vi "UI_update_Zone_indicator_params.vi"(8 "error in (no error)":errorcluster, 10 "Geometry params in":T1 {"Cage diameter, mm" scale=0.0..340.0}, 11 "Zone indicator ref. in":refnum<vi>) -> (0 "error out":errorcluster, 3 "Zone indicator ref. out":refnum<vi>)   [LabVIEW 2018, in "Tracker.lvlib"]
uses:
  Tracker.lvlib
  Controls/CTL_Segmented_plot_parameters.ctl
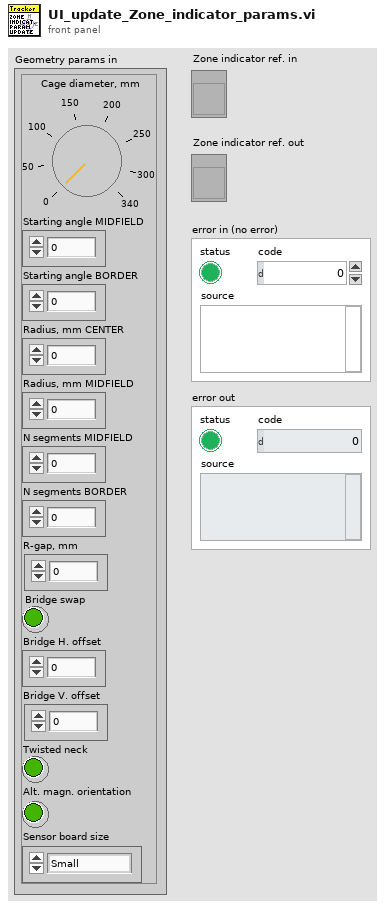
[diagram p1: front panel]
types:
  T1 = typedef "Tracker.lvlib/CTL_Segmented_plot_parameters.ctl" = cluster{"Cage diameter, mm":u16, "Starting angle MIDFIELD":i16, "Starting angle BORDER":i16, "Radius, mm CENTER":u16, "Radius, mm MIDFIELD":u16, "N segments MIDFIELD":u8, "N segments BORDER":u8, "R-gap, mm":sgl, "Bridge swap":bool, "Bridge H. offset":sgl, "Bridge V. offset":sgl, "Twisted neck":bool, "Alt. magn. orientation":bool, "Sensor board size":enum16{"Small", "Large"}}
  T2 = enum8{"Enabled", "Disabled", "Disabled and Grayed Out"}
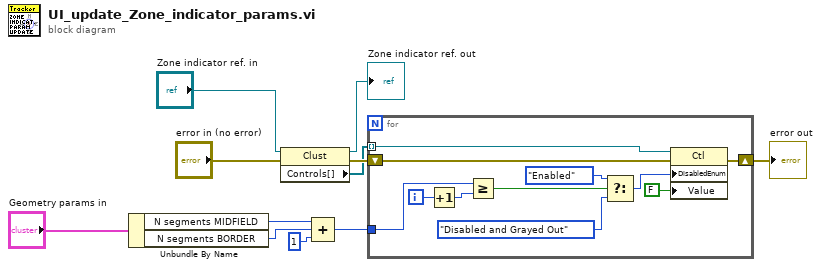
[diagram p0: block diagram]
diagram:
  n1 = Unbundle By Name("Geometry params in") -> ("N segments MIDFIELD"=w7:u8, "N segments BORDER"=w8:u8)
  n2 = property class="Clust"(reference="Zone indicator ref. in", error in="error in (no error)") -> (reference out=→"Zone indicator ref. out":refnum<vi>, error out=w10:errorcluster, "Controls[]"=w4:refnum<vi>[])
  n3 = Compound Arithmetic op=ADD(w7, w8, u8 1 ("value")) -> (w9:u8)
  n4 = for {
    tunnel: w4 -> [w17] mode=indexing
    tunnel: w9 -> [w13]
    shift-right: [w15] -> w11
    shift-left: w10 -> [w16]
    i -> [w14]
    n5 = Increment(x=w14) -> (x+1=w19:i32)
    n6 = Greater Or Equal?(x=w13, y=w19) -> (x >= y?=w18:bool)
    n7 = Select(t=T2."Enabled" ("Disabled"), s=w18, f=T2."Disabled and Grayed Out") -> (s? t:f=w21:T2)
    n8 = property class="Ctl"(reference=w17, error in=w16, "DisabledEnum"=w21, "Value"=FALSE) -> (error out=w15:errorcluster)  [unwired: 1 out]
  }
  "error out" <- w11
